vi "TangoSelectPos.vi"(7 "TANGO ID":i32, 8 "error in (no error)":errorcluster, 9 "Button":string, 10 "ItemNames":string[][](array[string])) -> (0 "error out":errorcluster)   [LabVIEW 2018, in "TangoOWN.lvlib"]
uses:
  TangoOWN.lvlib
  SDK/Tango.lvlib
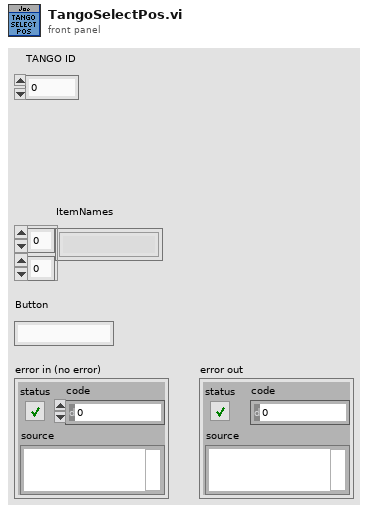
[diagram p1: front panel]
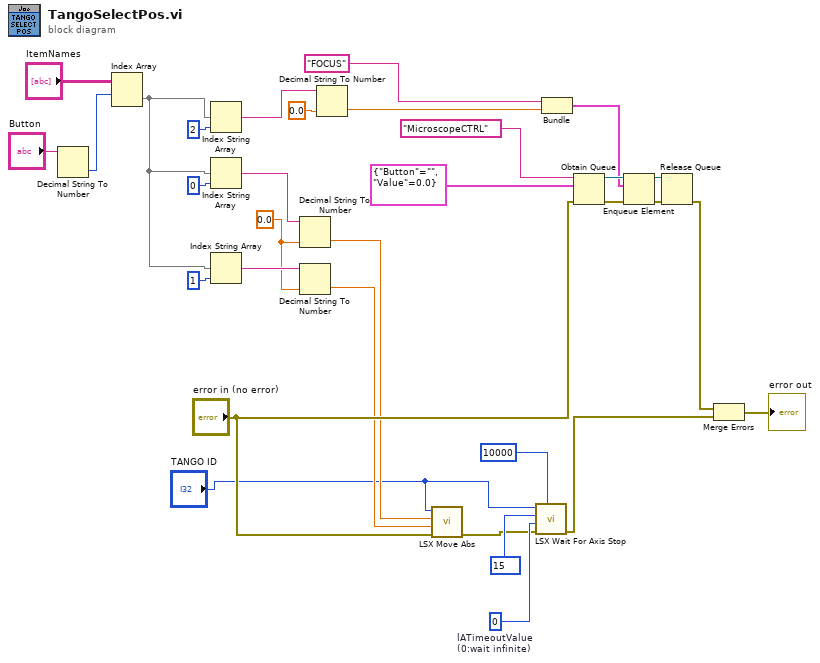
[diagram p0: block diagram]
diagram:
  w10 = 0  # lATimeoutValue (0:wait infinite)
  w18 = 0.0
  n1 = Decimal String To Number(string="Button") -> (number=w13:i32)  [unwired: 2 in, 1 out]
  n2 = Index Array(array="ItemNames", index (row)=w13) -> (element=w32:string[])  [unwired: 1 in]
  n3 = Index String Array(1:2 ("index"), 2:w32) -> (0:w22:string)  [unwired: 1 in]
  n4 = Index String Array(1:0 ("index"), 2:w32) -> (0:w17:string)  [unwired: 1 in]
  n5 = Index String Array(1:1 ("index"), 2:w32) -> (0:w20:string)  [unwired: 1 in]
  n6 = Decimal String To Number(string=w17, default (0L)=w18) -> (number=w19:dbl)  [unwired: 1 in, 1 out]
  n7 = Decimal String To Number(string=w20, default (0L)=w18) -> (number=w21:dbl)  [unwired: 1 in, 1 out]
  n8 = Decimal String To Number(string=w22, default (0L)=0.0 ("default (0 I32)")) -> (number=w26:dbl)  [unwired: 1 in, 1 out]
  n9 = call "LSX Move Abs.vi"("error in (no error)"="error in (no error)", "dY"=w21, "dX"=w19, "lLSID"="TANGO ID") -> ("error out"=w6:errorcluster)  [unwired: 6 in, 1 out]
  n10 = call "LSX Wait For Axis Stop.vi"("pbATimeout"=10000, "error in (no error)"=w6, "lATimeoutValue"=w10, "lAFlags"=i8 15, "lLSID"="TANGO ID") -> ("error out"=w1:errorcluster)  [unwired: 4 in, 2 out]
  n11 = Bundle("FOCUS", w26) -> (w27:cluster{string, dbl})  [unwired: 1 in]
  n12 = Obtain Queue(name (unnamed)="MicroscopeCTRL", element data type=cluster{"Button":string, "Value":dbl} {"Button"="", "Value"=0.0}, error in (no error)="error in (no error)") -> (queue out=w28:refnum<queue>, error out=w29:errorcluster)  [unwired: 2 in, 1 out]
  n13 = Enqueue Element(queue=w28, element=w27, error in (no error)=w29) -> (queue out=w4:refnum<queue>, error out=w3:errorcluster)  [unwired: 1 in, 1 out]
  n14 = Release Queue(queue=w4, error in (no error)=w3) -> (error out=w2:errorcluster)  [unwired: 1 in, 2 out]
  n15 = Merge Errors(w2, w1) -> (→"error out":errorcluster)
